vi "Write Config Data.vi"(8 "error in":errorcluster, 10 "Config Data":refnum<class "Data.lvclass">[](array[class]), 11 "Sequence Builder in":refnum<class "Sequence Builder.lvclass">) -> (0 "error out":errorcluster, 3 "Sequence Builder out":refnum<class "Sequence Builder.lvclass">)   [LabVIEW 2014, in "Sequence Builder.lvclass"]
uses:
  Sequence Builder.lvclass
  Data/Data.lvclass
  Sequence Builder.lvclass/Sequence Builder.ctl
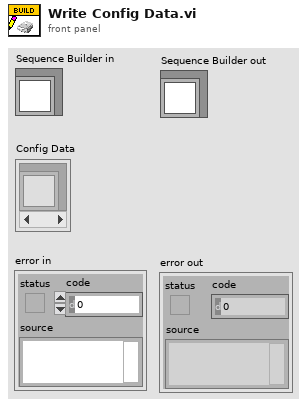
[diagram p1: front panel]
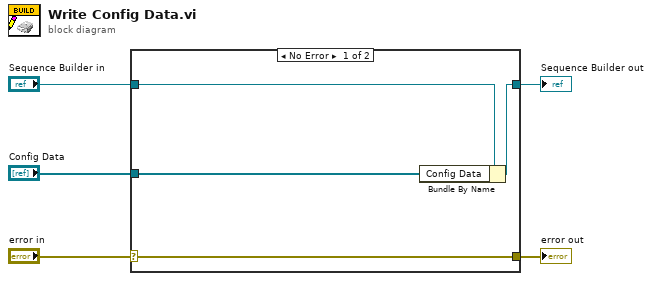
[diagram p0: block diagram]
diagram:
  n1 = case shown="No Error" "error in" {
    selector: "error in" -> [w9 w10]
    tunnel: [w9 w10] -> w4
    tunnel: [w7 w11] -> w2
    tunnel: "Sequence Builder in" -> [w8 w11]
    tunnel: "Config Data" -> [w6 _]
    frame No Error {
      n2 = Bundle By Name(cluster=w8, "Config Data"=w6) -> (w7:refnum<class "Sequence Builder.lvclass">)
    }
    frame Error {
    }
  }
  "error out" <- w4
  "Sequence Builder out" <- w2
